vi "thermo_get_format_strings.vi"(4 "format prefix":string, 5 "type index":T1) -> (0 "format strings":string[](array[string]), 1 "pres format":string, 2 "RH format":string, 3 "temp format":string)   [LabVIEW 2020]
uses:
  thermo_types.ctl
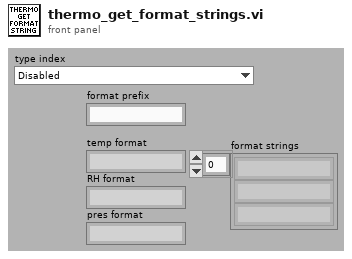
[diagram p1: front panel]
types:
  T1 = typedef "thermo_types.ctl" = enum16{"Disabled", "Simulated", "COMET Tx5xx (ethernet)", "Keithley 2002 (GPIB) + RTD", "Agilent 344xx (GPIB) + RTD"}
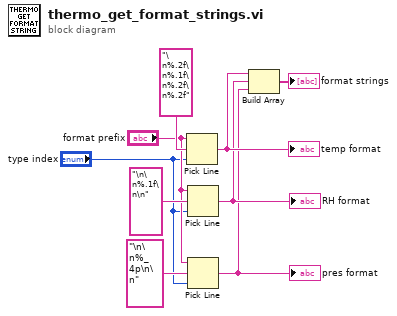
[diagram p0: block diagram]
diagram:
  n1 = Pick Line(string ("")="format prefix", multi-line string="\n%.2f\n%.1f\n%.2f\n%.2f", line index="type index") -> (output string=w6:string)
  "temp format" <- w6
  n2 = Pick Line(string ("")="format prefix", multi-line string="\n\n%.1f\n\n", line index="type index") -> (output string=w5:string)
  "RH format" <- w5
  n3 = Pick Line(string ("")="format prefix", multi-line string="\n\n%_4p\n\n", line index="type index") -> (output string=w4:string)
  "pres format" <- w4
  n4 = Build Array(w6, w5, w4) -> (→"format strings":string[])
